vi "2DMathPlot Action String.vi"(11 "Global String":T1 items=["Show/Hide", "Change Attribute", "Text Edit", "Cursor Move"]) -> (3 "String Out":string)   [LabVIEW 2017]
uses:
  <vilib>/Math Plots/2D Math Plots/2D Plot/Action String/2DMathPlot Action String.ctl
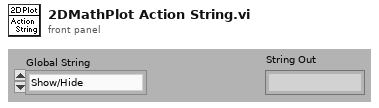
[diagram p1: front panel]
types:
  T1 = typedef "2DMathPlot Action String.ctl" = u16
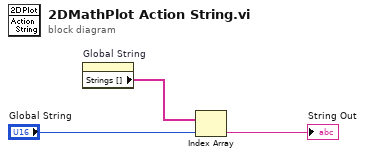
[diagram p0: block diagram]
diagram:
  n1 = property on="Global String" class="Ring (strict)"() -> ("Strings []"=w3:string[])  [unwired: 2 in, 2 out]
  n2 = Index Array(array=w3, index="Global String") -> (element=→"String Out":string)
